vi "Launch Data Viewer.vi"(8 "error in (no error)":errorcluster, 9 "stop pointer":refnum<class "Pointer.lvclass">, 11 "Server IP Address (localhost)":string="localhost") -> (0 "error out":errorcluster)   [LabVIEW 2019, in "DSF Core.lvlib"]
uses:
  DSF Core.lvlib
  <vilib>/NI/Memory Manager/Classes/Pointer/Pointer.lvclass
  Data Viewer.vi
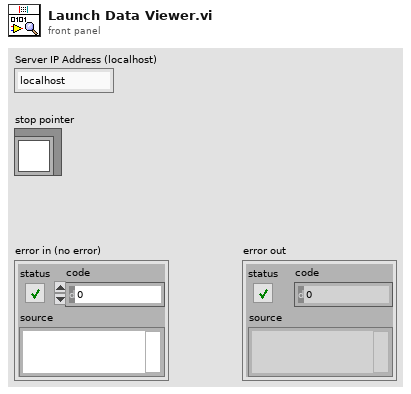
[diagram p1: front panel]
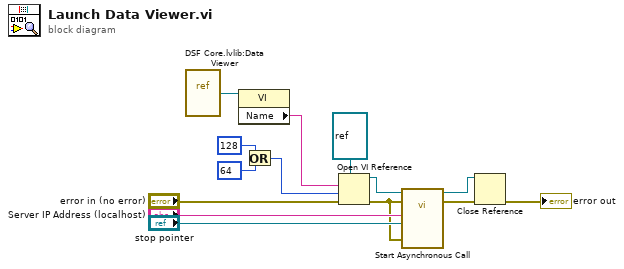
[diagram p0: block diagram]
diagram:
  n1 = vi-ref "DSF Core.lvlib:Data Viewer.vi"() -> (w7:refnum<vi>)
  n2 = property class="VI"(reference=w7) -> ("Name"=w6:string)  [unwired: 1 in, 2 out]
  n3 = Or(x=128 ("options"), y=64 ("options")) -> (x .or. y?=w3:i32)
  n4 = Open VI Reference(type specifier VI Refnum (for type only)=refnum<vi> refnum, vi path=w6, options=w3, error in (no error)="error in (no error)") -> (vi reference=w4:refnum<vi>, error out=w10:errorcluster)  [unwired: 2 in]
  n5 = call-by-ref "Start Asynchronous Call"(reference=w4, error in=w10, 8:"error in (no error)"=w10, "stop pointer"="stop pointer", "Server IP Address"="Server IP Address (localhost)") -> (reference out=w1:refnum<vi>, error out=w2:errorcluster)  [unwired: 8 in, 1 out]
  n6 = Close Reference(reference=w1, error in (no error)=w2) -> (error out=→"error out":errorcluster)
